vi "N5232-PNA_ListShortcuts.vi"(0 "Session In":refnum<visa-resource-name>="TCPIP0::169.254.70.180::inst0::INSTR", 11 "error in":errorcluster {"code" format="%.0x"}, 13 "ShortcutNum":string) -> (2 "shortcut(ary)":string[](array[string])=["\"Pulse\"", "\"AdaptorChar\"", "\"MapZ\"", "\"\"", "\"\"", "\"\"", "\"\"", "\"\"", "\"\"", "\"\"", "\"\"", "\"\"", "\"\"", "\"\"", "\"\"", "\"\"", "\"\"", "\"\"", "\"\"", "\"\"", "\"\"", "\"\"", "\"\"", "\"\"", "\"\""], 3 "shortcut":string="\"\"", 4 "Session Out":refnum<visa-resource-name>="TCPIP0::169.254.70.180::inst0::INSTR", 15 "error out":errorcluster {"code" format="%.0x"})   [LabVIEW 2018]
doc: "Launches the Instrument I/O Assistant, which you can use to communicate with message-based instruments and graphically parse the response. For example you can communicate with an instrument that uses a serial, Ethernet, or GPIB interface."
panel:
  # "Shortcuts on N5232A are also known as \"Macros\" listed in the UTILITY menu"
  # "Enter a number 1-25. Leave Blank or write \"ALL\" to get the list of all available shortcuts"
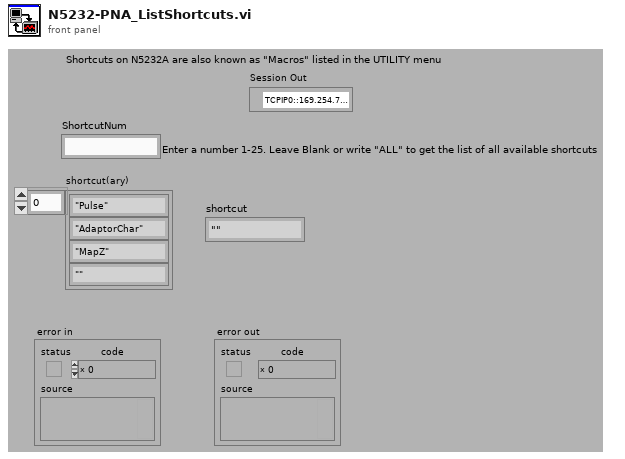
[diagram p1: front panel]
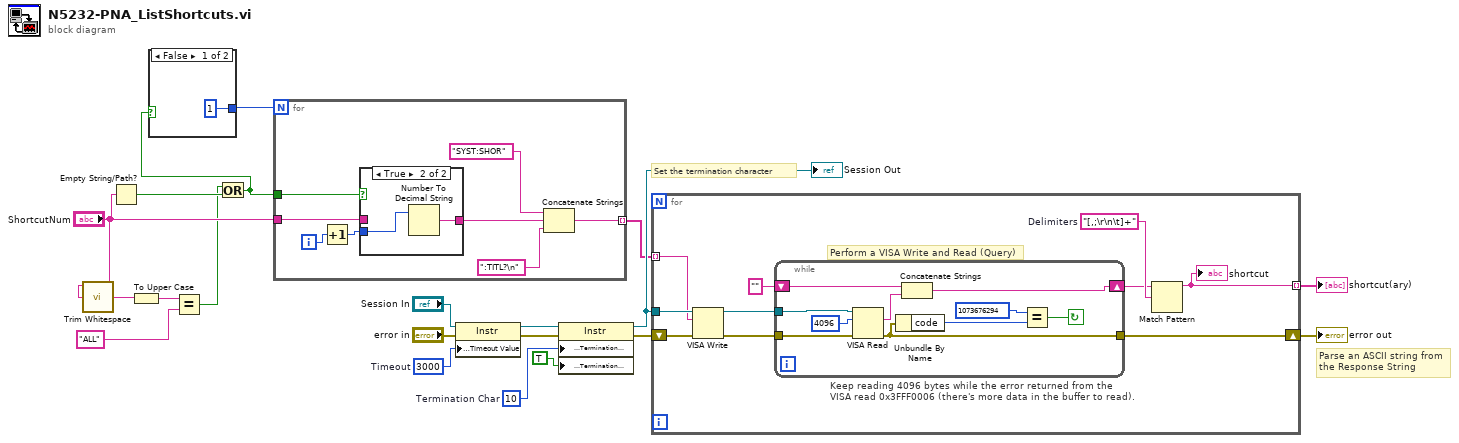
[diagram p0: block diagram]
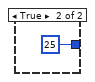
[diagram p2: hidden frame]
diagram:
  w15 = u8 10  # Termination Char
  w20 = u32 3000  # Timeout
  # "Parse an ASCII string from the Response String"
  # "Set the termination character"
  n1 = call <vilib>:"Trim Whitespace.vi"("string"="ShortcutNum") -> ("trimmed string"=w6:string)  [unwired: 1 in]
  n2 = Empty String/Path?(string/path="ShortcutNum") -> (empty?=w7:bool)
  n3 = To Upper Case(1:w6) -> (0:w4:string)
  n4 = Equal?(x=w4, y="ALL") -> (x = y?=w2:bool)
  n5 = Or(x=w2, y=w7) -> (x .or. y?=w1:bool)
  n6 = case shown="False" w1 {
    tunnel: [1 25] -> w8
    frame False {
    }
    frame True {
    }
  }
  n7 = for {
    N: w8 -> [_]
    tunnel: [w28] -> w9 mode=indexing
    tunnel: "ShortcutNum" -> [w26]
    tunnel: w1 -> [w25]
    i -> [w30]
    n8 = Increment(x=w30) -> (x+1=w29:i32)
    n9 = case shown="True" w25 {
      tunnel: w29 -> [_ w33]
      tunnel: [w31 w32] -> w27
      tunnel: w26 -> [w31 _]
      frame False {
      }
      frame True {
        n10 = Number To Decimal String(number=w33) -> (decimal integer string=w32:string)  [unwired: 1 in]
      }
    }
    n11 = Concatenate Strings("SYST:SHOR" ("Command"), w27, ":TITL?\n" ("Command")) -> (w28:string)
  }
  n12 = property class="Instr"(reference="Session In", error in="error in", "General Settings:Timeout Value"=w20) -> (reference out=w14:refnum<visa-resource-name>, error out=w17:errorcluster)
  n13 = property class="Instr"(reference=w14, error in=w17, "Message Based Settings:Termination Character"=w15, "Message Based Settings:Termination Character Enable"=TRUE ("enable")) -> (reference out=w10:refnum<visa-resource-name>, error out=w16:errorcluster)
  "Session Out" <- w10
  n14 = for {
    tunnel: [w38] -> w11 mode=indexing
    tunnel: w10 -> [w35]
    tunnel: w9 -> [w34] mode=indexing
    shift-right: [w40] -> w12
    shift-left: w16 -> [w43]
    w37 = "[,;\r\n\t]+"  # Delimiters
    # "Perform a VISA Write and Read (Query)"
    # "Keep reading 4096 bytes while the error returned from the\nVISA read 0x3FFF0006 (there's more data in the buffer to read)."
    n15 = VISA Write(VISA resource name=w35, write buffer=w34, error in (no error)=w43) -> (VISA resource name out=w42:refnum<visa-resource-name>, error out=w41:errorcluster)  [unwired: 1 out]
    n16 = while {
      tunnel: w42 -> [w50]
      shift-right: [w44] -> w36
      shift-left: "" -> [w49]
      tunnel: w41 -> [w47]
      tunnel: [w46] -> w40
      stop <- w45 continue-if-true
      n17 = VISA Read(VISA resource name=w50, byte count=u32 4096 ("byte count (0)"), error in (no error)=w47) -> (read buffer=w48:string, error out=w46:errorcluster)  [unwired: 2 out]
      n18 = Unbundle By Name(w46) -> ("code"=w52:i32)
      n19 = Concatenate Strings(w49, w48) -> (w44:string)
      n20 = Equal?(x=1073676294, y=w52) -> (x = y?=w45:bool)
    }
    n21 = Match Pattern(string=w36, regular expression=w37) -> (before substring=w38:string)  [unwired: 4 out]
    "shortcut" <- w38
  }
  "shortcut(ary)" <- w11
  "error out" <- w12
